vi "Read Base Actor DVR.vi"(11 "Base Actor in":refnum<class "Base Actor.lvclass">) -> (2 "Base Actor DVR":refnum<data-value>)   [LabVIEW 2020, in "jettl.lvlib" / "Base jettl Actor.lvlib" / "Base Actor.lvlib" / "Base Actor.lvclass"]
uses:
  Base Actor.lvclass
  Base Actor.lvclass/Base Actor.ctl
  Msg/Msg.lvclass
  Unified Actor Lifetime.ctl
  jettl.lvlib
  Base Actor.ctl
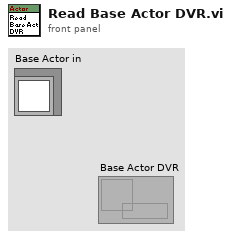
[diagram p1: front panel]
types:
  T1 = typedef "jettl.lvlib/Base Actor.ctl" = cluster{"Unified Actor Lifetime":T2, "Msg DVR":refnum<data-value>}
  T2 = typedef "jettl.lvlib/Unified Actor Lifetime.ctl" = enum16{"Init", "Spawn", "Setup", "Teardown Before Running", "Running", "Stop Called", "Stopping With Children", "Stopping Without Children", "Teardown After Running", "Stopped"}
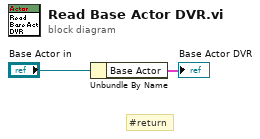
[diagram p0: block diagram]
diagram:
  # "#return"
  n1 = Unbundle By Name("Base Actor in") -> ("Base Actor"=→"Base Actor DVR":T1)
